vi "Read out ISET.vi"(4 "get more?":bool, 5 "All Channels (T)":bool=TRUE, 7 "Channel":u8, 8 "error in (no error)":errorcluster, 11 "BoardHandle":T2) -> (0 "error out":errorcluster, 1 "ISet constants":T1(array[cluster]), 2 "ISet values (uA)":dbl[](array[numeric]), 3 "BoardHandle out":T2)   [LabVIEW 2020, in "CAEN PSM.lvlib"]
doc: "This function returns Iset value"
uses:
  CAEN PSM.lvlib
  Private/BoardHandle.ctl
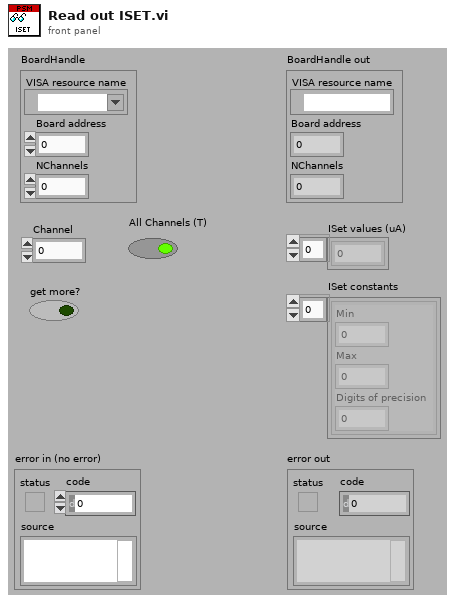
[diagram p1: front panel]
types:
  T1 = cluster{"Min":dbl, "Max":dbl, "Digits of precision":i32}[]
  T2 = typedef "CAEN PSM.lvlib/BoardHandle.ctl" = cluster{"VISA resource name":refnum<visa-resource-name>, "Board address":i8, "NChannels":u8}
  T3 = cluster{"Min":dbl, "Max":dbl, "Digits of precision":i32}
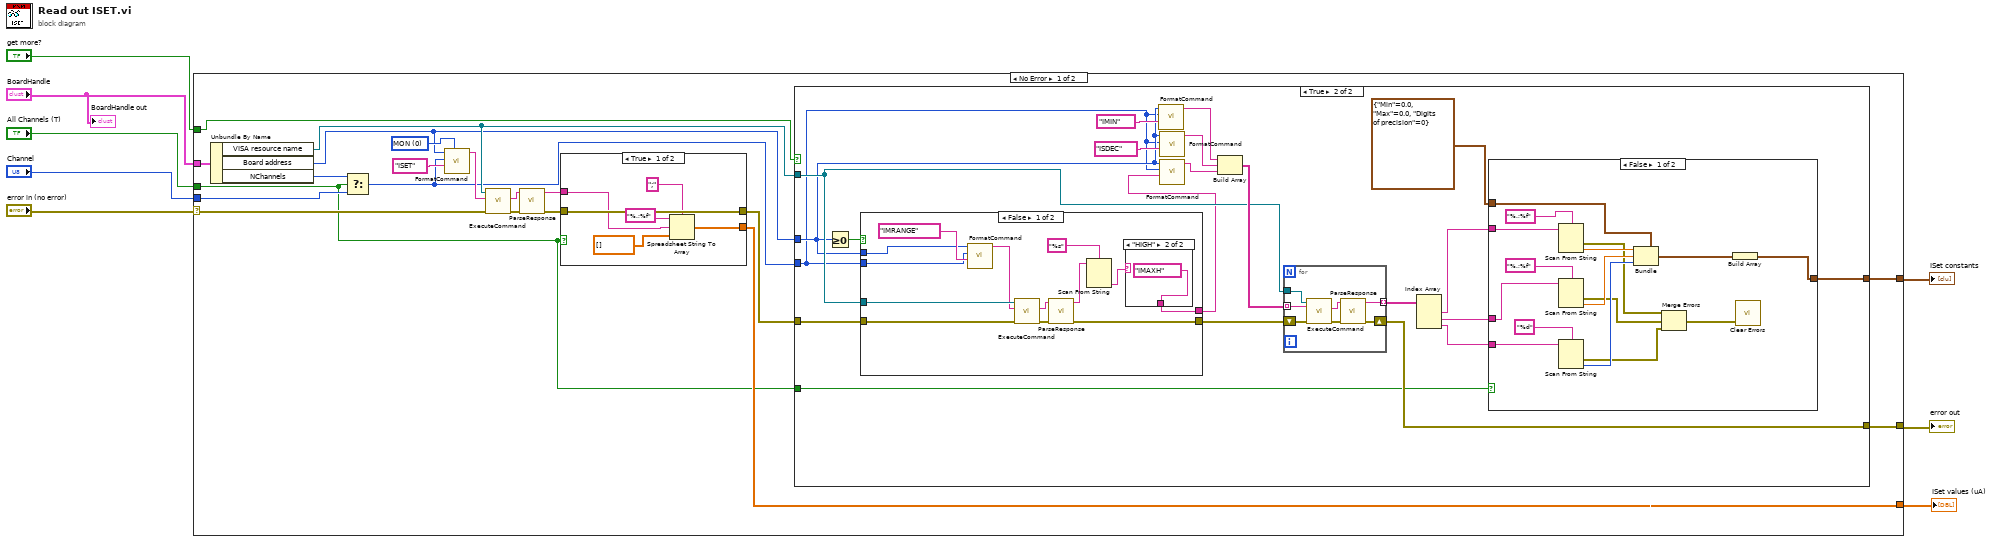
[diagram p0: block diagram]
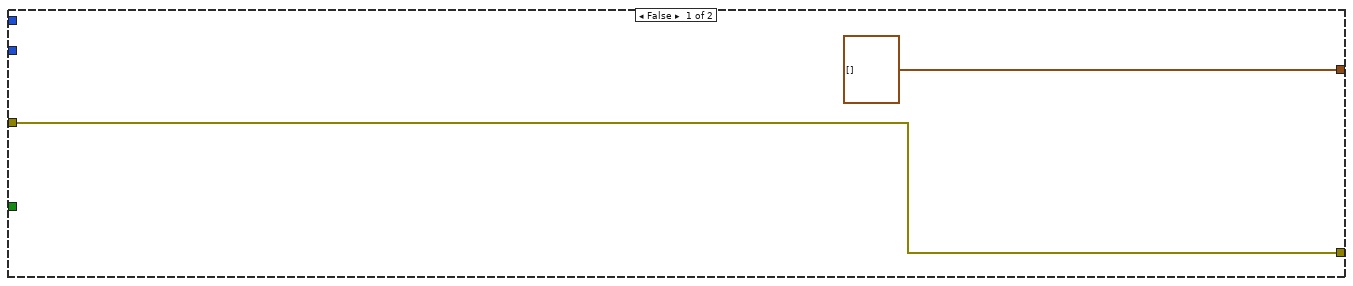
[diagram p2: hidden frame]
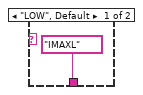
[diagram p3: hidden frame]
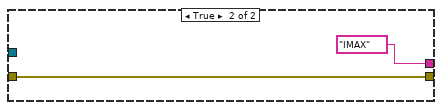
[diagram p4: hidden frame]
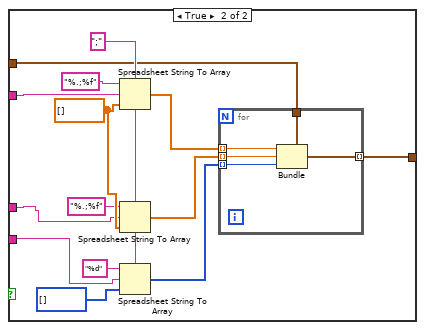
[diagram p5: hidden frame]
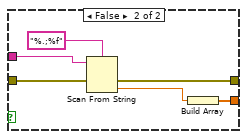
[diagram p6: hidden frame]
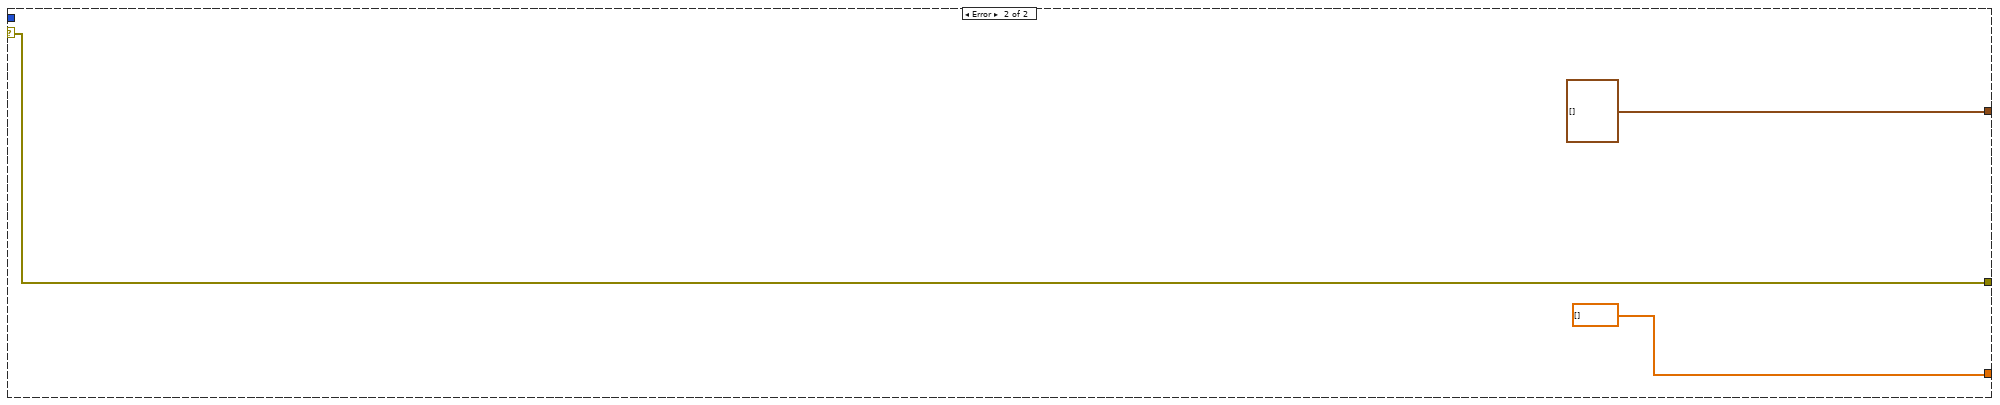
[diagram p7: hidden frame]
diagram:
  n1 = case shown="No Error" "error in (no error)" {
    selector: "error in (no error)" -> [w22 w125]
    tunnel: "All Channels (T)" -> [w9 _]
    tunnel: "Channel" -> [w27 _]
    tunnel: [w12 w125] -> w5
    tunnel: "BoardHandle" -> [w23 _]
    tunnel: [w17 dbl[] [] ("Trip value(s) s")] -> w3
    tunnel: "get more?" -> [w16 _]
    tunnel: [w11 T1 []] -> w1
    frame No Error {
      w28 = u8 0 items=["MON", "SET"] ("CMD")
      n2 = Unbundle By Name(w23) -> ("VISA resource name"=w15:refnum<visa-resource-name>, "Board address"=w10:i8, "NChannels"=w20:u8)
      n3 = Select(t=w20, s=w9, f=w27) -> (s? t:f=w14:u8)
      n4 = call "FormatCommand.vi"("CMD (MON)"=w28, "PAR"="ISET", "CH"=w14, "BD (0)"=w10) -> ("cmd"=w26:string)  [unwired: 7 in]
      n5 = call "ExecuteCommand.vi"("error in (no error)"=w22, "Command"=w26, "VISA resource name"=w15) -> ("error out"=w25:errorcluster, "Response"=w24:string)  [unwired: 6 in, 1 out]
      n6 = call "ParseResponse.vi"("error in (no error)"=w25, "Response"=w24) -> ("error out"=w18:errorcluster, "val"=w19:string)  [unwired: 6 in, 2 out]
      n7 = case shown="True" w9 {
        tunnel: w19 -> [w111 w122]
        tunnel: w18 -> [w116 w120]
        tunnel: [w116 w119] -> w13
        tunnel: [w112 w117] -> w17
        frame True {
          n8 = Spreadsheet String To Array(delimiter (Tab)=";", format string="%.;%f", spreadsheet string=w111, array type (2D Dbl)=dbl[] []) -> (array=w112:dbl[])
        }
        frame False {
          n9 = Scan From String(format string="%.;%f", input string=w122, error in=w120) -> (error out=w119:errorcluster, output 1=w118:dbl)  [unwired: 2 in, 2 out]
          n10 = Build Array(w118) -> (w117:dbl[])
        }
      }
      n11 = case shown="True" w16 {
        tunnel: w13 -> [w30 w40]
        tunnel: [w30 w49] -> w12
        tunnel: w15 -> [_ w34]
        tunnel: w10 -> [_ w32]
        tunnel: w14 -> [_ w31]
        tunnel: [T1 [] w44] -> w11
        tunnel: w9 -> [_ w43]
        frame False {
        }
        frame True {
          n12 = Greater Or Equal To 0?(x=w32) -> (x >= 0?=w41:bool)
          n13 = case shown="False" w41 {
            tunnel: w40 -> [w61 w68]
            tunnel: [w60 w68] -> w39
            tunnel: w34 -> [w59 _]
            tunnel: w32 -> [w57 _]
            tunnel: w31 -> [w56 _]
            tunnel: [w52 "IMAX" ("PAR")] -> w33
            frame False {
              n14 = call "FormatCommand.vi"("PAR"="IMRANGE", "CH"=w56, "BD (0)"=w57) -> ("cmd"=w58:string)  [unwired: 8 in]
              n15 = call "ExecuteCommand.vi"("error in (no error)"=w61, "Command"=w58, "VISA resource name"=w59) -> ("error out"=w63:errorcluster, "Response"=w62:string)  [unwired: 6 in, 1 out]
              n16 = call "ParseResponse.vi"("error in (no error)"=w63, "Response"=w62) -> ("error out"=w60:errorcluster, "val"=w54:string)  [unwired: 6 in, 2 out]
              n17 = Scan From String(format string="%s", input string=w54) -> (output 1=w53:string)  [unwired: 3 in, 3 out]
              n18 = case shown="\"HIGH\"" w53 {
                tunnel: ["IMAXL" ("PAR") "IMAXH" ("PAR")] -> w52
                frame "LOW", Default {
                }
                frame "HIGH" {
                }
              }
            }
            frame True {
            }
          }
          n19 = call "FormatCommand.vi"("PAR"="IMIN", "CH"=w31, "BD (0)"=w32) -> ("cmd"=w37:string)  [unwired: 8 in]
          n20 = call "FormatCommand.vi"("PAR"="ISDEC", "CH"=w31, "BD (0)"=w32) -> ("cmd"=w36:string)  [unwired: 8 in]
          n21 = call "FormatCommand.vi"("PAR"=w33, "CH"=w31, "BD (0)"=w32) -> ("cmd"=w38:string)  [unwired: 8 in]
          n22 = Build Array(w37, w36, w38) -> (w35:string[])
          n23 = for {
            shift-right: [w109] -> w49
            shift-left: w39 -> [w110]
            tunnel: [w106] -> w48 mode=indexing
            tunnel: w35 -> [w105] mode=indexing
            tunnel: w34 -> [w104]
            n24 = call "ExecuteCommand.vi"("error in (no error)"=w110, "Command"=w105, "VISA resource name"=w104) -> ("error out"=w108:errorcluster, "Response"=w107:string)  [unwired: 6 in, 1 out]
            n25 = call "ParseResponse.vi"("error in (no error)"=w108, "Response"=w107) -> ("error out"=w109:errorcluster, "val"=w106:string)  [unwired: 6 in, 2 out]
          }
          n26 = Index Array(array=w48) -> (element #1=w47:string, element #2=w46:string, element #3=w45:string)  [unwired: 3 in]
          n27 = case shown="False" w43 {
            tunnel: w47 -> [w84 w85]
            tunnel: w46 -> [w79 w86]
            tunnel: w45 -> [w80 w87]
            tunnel: T3 {"Min"=0.0, "Max"=0.0, "Digits of precision"=0} -> [w78 w89]
            tunnel: [w73 w88] -> w44
            frame False {
              n28 = Scan From String(format string="%.;%f", input string=w84) -> (error out=w72:errorcluster, output 1=w77:dbl)  [unwired: 3 in, 2 out]
              n29 = Scan From String(format string="%.;%f", input string=w79) -> (error out=w71:errorcluster, output 1=w76:dbl)  [unwired: 3 in, 2 out]
              n30 = Scan From String(format string="%d", input string=w80) -> (error out=w70:errorcluster, output 1=w75:i32)  [unwired: 3 in, 2 out]
              n31 = Bundle(cluster=w78, "Min"=w77, "Max"=w76, "Digits of precision"=w75) -> (w74:T3)
              n32 = Merge Errors(w72, w71, w70) -> (w69:errorcluster)
              n33 = Build Array(w74) -> (w73:T1)
              n34 = call <vilib>:"Clear Errors.vi"("error in (no error)"=w69) -> ()  [unwired: 5 in, 2 out]
            }
            frame True {
              w94 = dbl[] [] ("array type (2D Dbl)")
              w93 = ";" ("delimiter (Tab)")
              n35 = Spreadsheet String To Array(delimiter (Tab)=w93, format string="%.;%f", spreadsheet string=w85, array type (2D Dbl)=w94) -> (array=w96:dbl[])
              n36 = Spreadsheet String To Array(delimiter (Tab)=w93, format string="%.;%f", spreadsheet string=w86, array type (2D Dbl)=w94) -> (array=w97:dbl[])
              n37 = Spreadsheet String To Array(delimiter (Tab)=w93, format string="%d", spreadsheet string=w87, array type (2D Dbl)=i32[] []) -> (array=w98:i32[])
              n38 = for {
                tunnel: w89 -> [w103]
                tunnel: w96 -> [w102] mode=indexing
                tunnel: w97 -> [w100] mode=indexing
                tunnel: w98 -> [w101] mode=indexing
                tunnel: [w99] -> w88 mode=indexing
                n39 = Bundle(cluster=w103, "Min"=w102, "Max"=w100, "Digits of precision"=w101) -> (w99:T3)
              }
            }
          }
        }
      }
    }
    frame Error {
    }
  }
  "error out" <- w5
  "ISet values (uA)" <- w3
  "ISet constants" <- w1
  "BoardHandle out" <- "BoardHandle"
